vi "FTW-Endpoint-Connect.vi"(0 "FTW Socket":refnum<class "FTW-Actor-Endpoint.lvclass">, 5 "Remote Address":string, 11 "error in":errorcluster) -> (4 "FTW Socket out":refnum<class "FTW-Actor-Endpoint.lvclass">, 15 "error out":errorcluster)   [LabVIEW 2013, in "FTW-Actor-Endpoint.lvclass"]
uses:
  FTW-Actor-Endpoint.lvclass
  FTW-Actor-Endpoint.lvclass/FTW-Actor-Endpoint.ctl
panel:
  # "Inputs"
  # "Outputs"
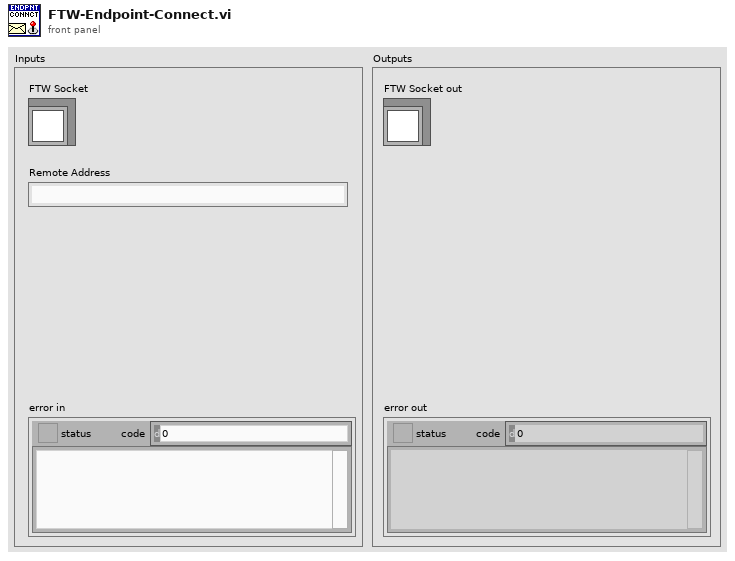
[diagram p1: front panel]
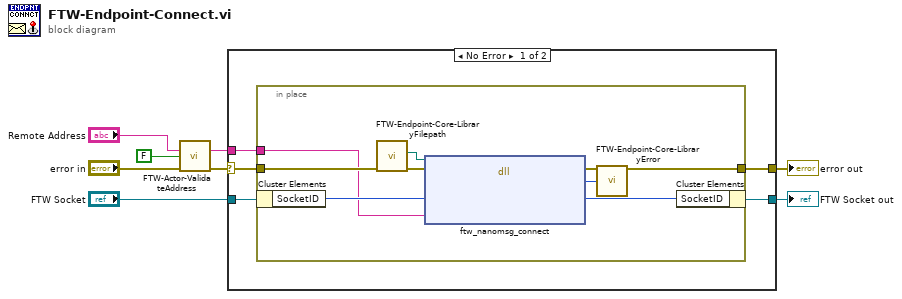
[diagram p0: block diagram]
diagram:
  n1 = call "FTW-Actor-ValidateAddress.vi"("Address"="Remote Address", "Allow wildcard replacement?"=FALSE, "error in"="error in") -> ("Sanitized Address"=w2:string, "error out"=w4:errorcluster)  [unwired: 10 in, 1 out]
  n2 = case shown="No Error" w4 {
    selector: w4 -> [w11 w23]
    tunnel: "FTW Socket" -> [w13 w24]
    tunnel: [w9 w23] -> w7
    tunnel: [w12 w24] -> w6
    tunnel: w2 -> [w10 _]
    frame No Error {
      n3 = in-place {
        in-place-border: w11 -> [w21]
        in-place-border: [w15] -> w9
        in-place-border: w10 -> [w20]
        n4 = in-place-cluster #1(w13) -> ("SocketID"=w22:i64)
        n5 = call "FTW-Endpoint-Core-LibraryFilepath.vi"("error in"=w21) -> ("error out"=w18:errorcluster, "Library Filepath"=w17:path)  [unwired: 8 in, 1 out]
        n6 = dll-call lib="?" fn="ftw_nanomsg_connect"(path in=w17, error in=w18, "SocketID"=w22, "Address"=w20) -> (error out=w16:errorcluster, "Return Value"=w14:i64, "SocketID"=w19:i64)  [unwired: 2 in, 1 out]
        n7 = call "FTW-Endpoint-Core-LibraryError.vi"("error in"=w16, "Return Value"=w14) -> ("error out"=w15:errorcluster)  [unwired: 13 in]
        n8 = in-place-cluster #1("SocketID"=w19) -> (w12:refnum<class "FTW-Actor-Endpoint.lvclass">)
      }
    }
    frame Error {
    }
  }
  "error out" <- w7
  "FTW Socket out" <- w6
